vi "DAQ_System.vi"() -> ()   [LabVIEW 2023]
uses:
  Controls/Control 5.ctl
  Controls/Control 4.ctl
  Controls/Queue_Operation_Select.ctl
  Controls/Acquired_Data.ctl
  Controls/State_and_Data.ctl
panel:
  out "Error_Out":errorcluster
  in  "Error_In":errorcluster
  in  "Stop":bool
  out "DAQ_Output":T1
  in  "DAQ_Inputs":T2 caption="DAQ Inputs" {"Analog_In"."Battery_Power" scale=0.0..10.0; "Analog_In"."Power_Consumption" scale=0.0..10.0}
  # "DAQ Simulator"
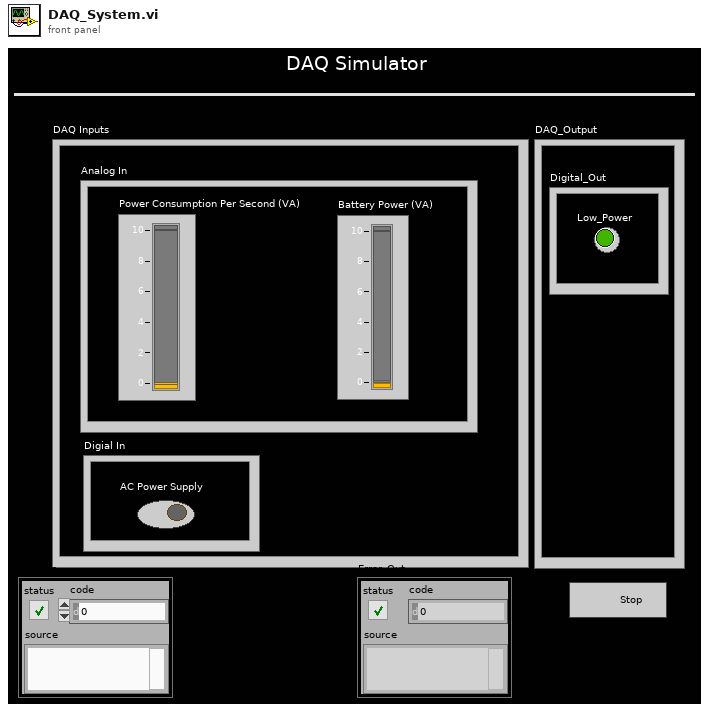
[diagram p1: front panel]
types:
  T1 = typedef "Control 4.ctl" = cluster{"Digital_Out":cluster{"Low_Power":bool}}
  T2 = typedef "Control 5.ctl" = cluster{"Digial_In":cluster{"AC_Power_Supply":bool}, "Analog_In":cluster{"Power_Consumption":dbl, "Battery_Power":dbl}}
  T3 = typedef "Acquired_Data.ctl" = cluster{"Battery_Power":dbl, "Power_Consumption":dbl, "Inverter_Mode":bool}
  T4 = typedef "State_and_Data.ctl" = cluster{"State":string, "Data":variant}
  T5 = cluster{"Low_Power?":bool, "Acquired_Data":T3, "DAQ_Output":T1, "DAQ_Inputs":T2, "Data_In":T4, "Start":bool}
  T6 = enum32{"Invalid", "Standard", "Closed", "Hidden", "Minimized", "Maximized"}
  T7 = typedef "Queue_Operation_Select.ctl" = enum16{"Obtain_Queue", "Enqueue", "Enqueue_First", "Enqueue_N", "Lossy_Enqueue", "Preview", "Queue_Status", "Dequeue", "Flush", "Release_Queue"}
  T8 = cluster{"Power_Consumption":dbl, "Battery_Power":dbl}
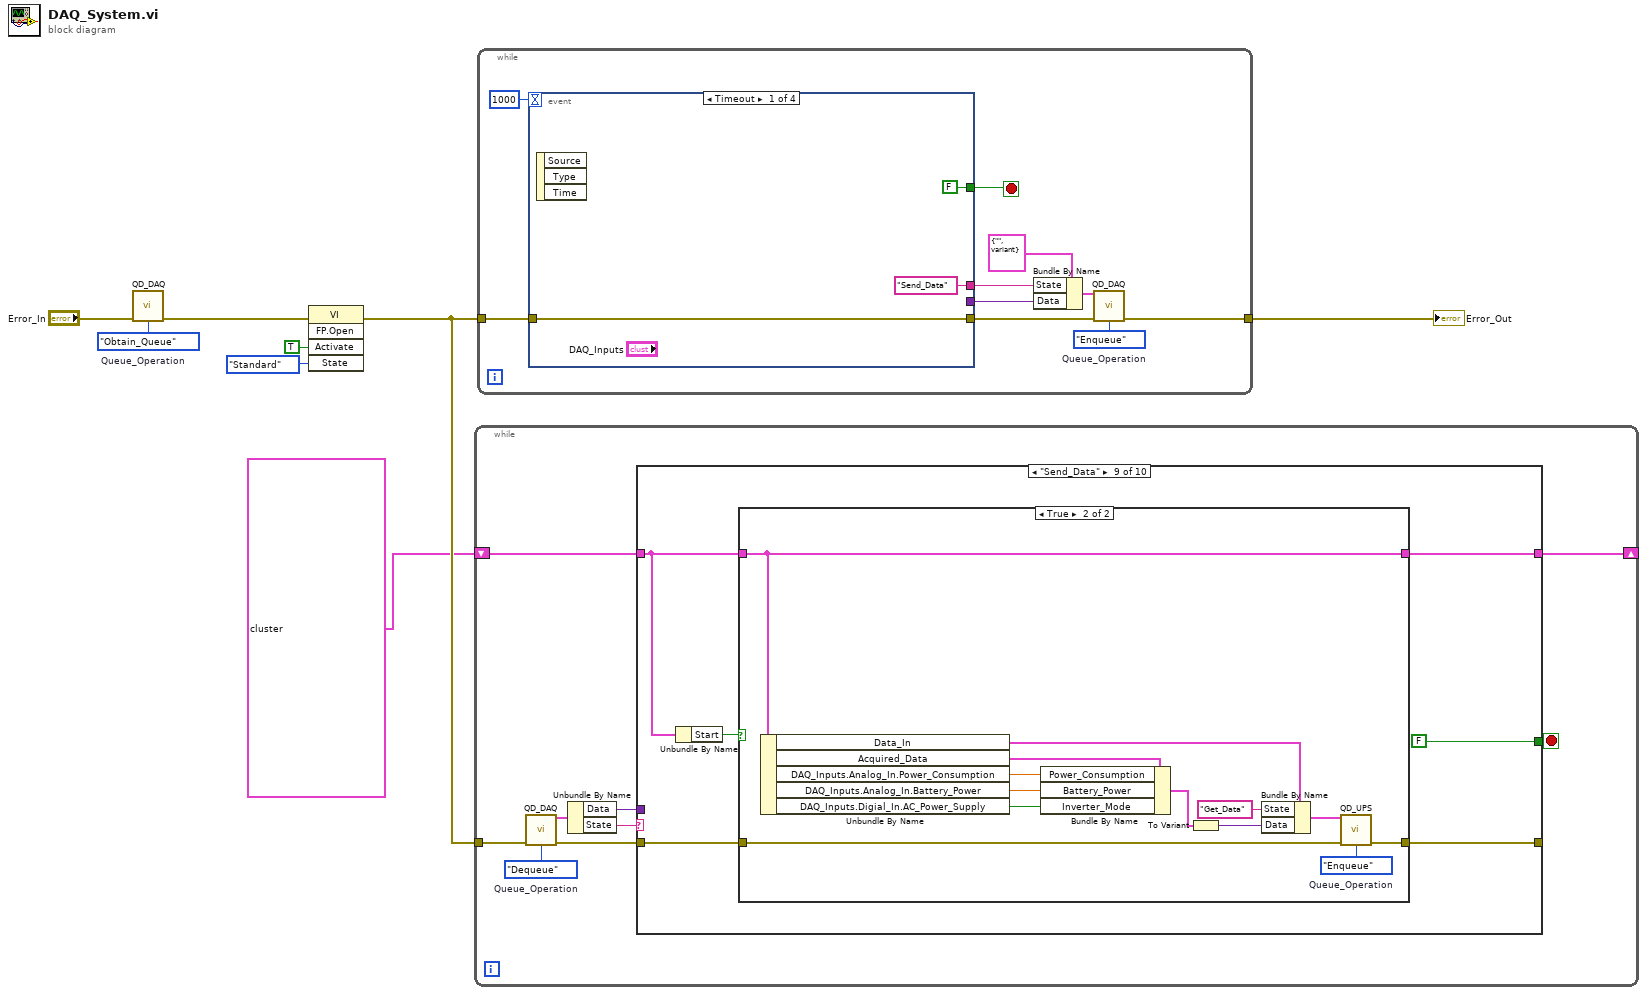
[diagram p0: block diagram]
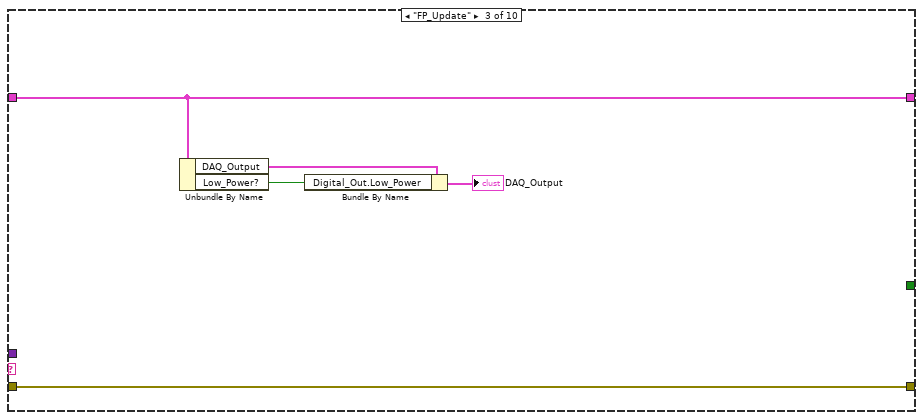
[diagram p4: hidden frame]
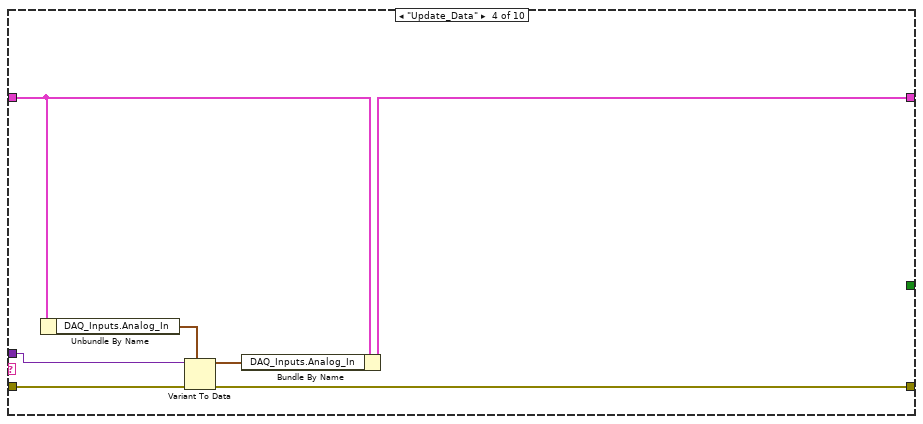
[diagram p5: hidden frame]
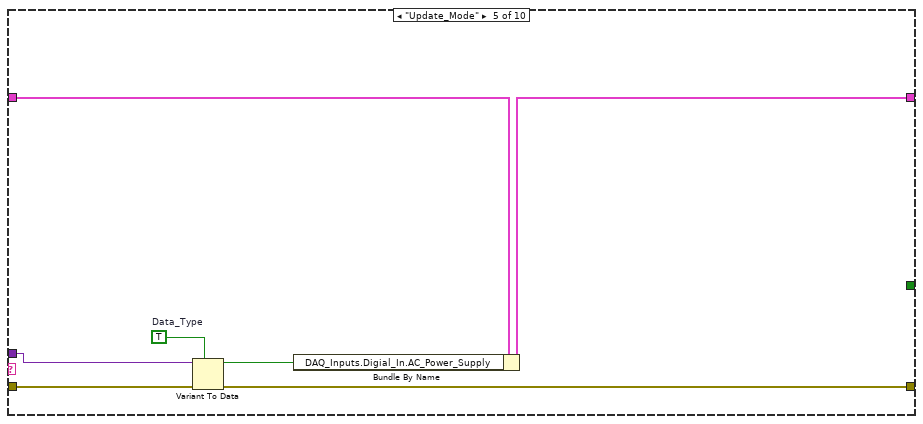
[diagram p6: hidden frame]
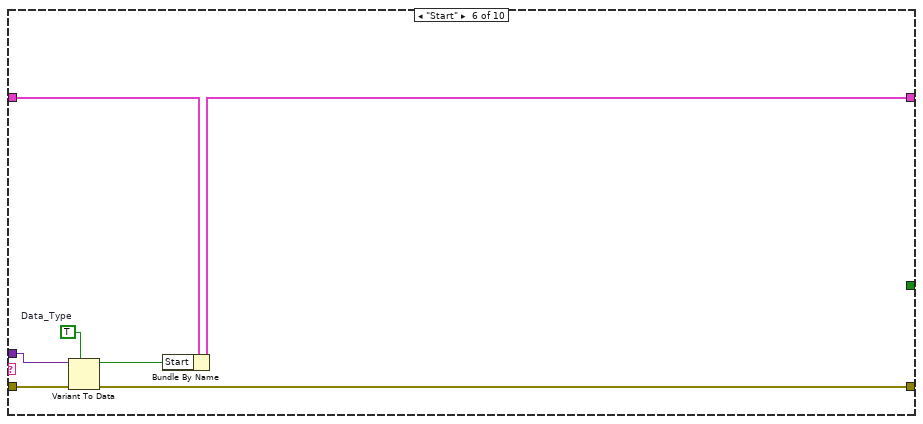
[diagram p7: hidden frame]
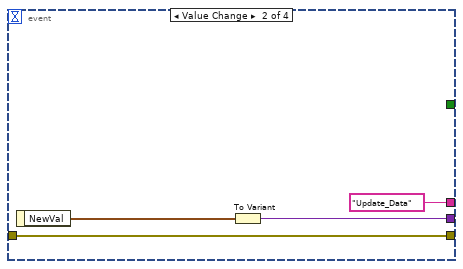
[diagram p12: hidden frame]
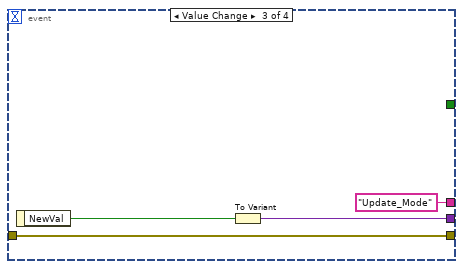
[diagram p13: hidden frame]
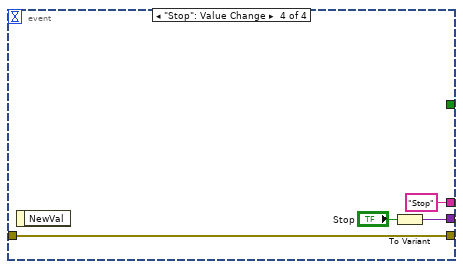
[diagram p14: hidden frame]
diagram:
  w5 = Queue_Operation_Select."Obtain_Queue"  # Queue_Operation
  n1 = call "QD_DAQ.vi"("Error_In"="Error_In", "Queue_Operation"=w5) -> ("Error_Out"=w6:errorcluster)  [unwired: 11 in, 2 out]
  n2 = invoke class="VI" method="FP.Open"(error in=w6, "Activate"=TRUE ("Activate?"), "State"=T6."Standard") -> (error out=w2:errorcluster)  [unwired: 2 in, 4 out]
  n3 = while {
    tunnel: w2 -> [w17]
    shift-right: [w11] -> _
    shift-left: T5 {"Low_Power?"=FALSE, "Acquired_Data"={"Battery_Power"=0.0, "Power_Consumption"=0.0, "Inverter_Mode"=FALSE}, "DAQ_Output"={"Digital_Out"={"Low_Power"=FALSE}}, "DAQ_Inputs"={"Digial_In"={"AC_Power_Supply"=FALSE}, "Analog_In"={"Power_Consumption"=0.0, "Battery_Power"=0.0}}, "Data_In"={"State"="", "Data"=variant}, "Start"=FALSE} -> [w10]
    stop <- w9 stop-if-true
    w15 = Queue_Operation_Select."Dequeue"  # Queue_Operation
    n4 = call "QD_DAQ.vi"("Error_In"=w17, "Queue_Operation"=w15) -> ("Data_Out"=w14:T4, "Error_Out"=w16:errorcluster)  [unwired: 11 in, 1 out]
    n5 = Unbundle By Name(w14) -> ("Data"=w12:variant, "State"=w13:string)
    n6 = case shown="\"Send_Data\"" w13 {
      tunnel: w16 -> [w19 w21 w26 w33 w40 w47 w49 w51 w57 w74]
      tunnel: [w19 w21 w26 w32 w39 w45 w49 w51 w56 w74] -> _
      tunnel: w12 -> [_ _ _ w31 w38 w44 _ _ _ _]
      tunnel: [w18 w20 w25 w28 w35 w42 w48 w50 w55 w73] -> w11
      tunnel: w10 -> [w18 w20 w25 w29 w37 w46 w48 w50 w54 w73]
      tunnel: [_ _ _ _ _ _ _ _ FALSE _] -> w9
      frame Default {
      }
      frame "Initialize" {
      }
      frame "FP_Update" {
        n7 = Unbundle By Name(w25) -> ("DAQ_Output"=w23:T1, "Low_Power?"=w22:bool)
        n8 = Bundle By Name(cluster=w23, "Digital_Out.Low_Power"=w22) -> (→"DAQ_Output":T1)
      }
      frame "Update_Data" {
        n9 = Unbundle By Name(w29) -> ("DAQ_Inputs.Analog_In"=w30:T8)
        n10 = Variant To Data(error in=w33, type=w30, Variant=w31) -> (data=w27:T8, error out=w32:errorcluster)
        n11 = Bundle By Name(cluster=w29, "DAQ_Inputs.Analog_In"=w27) -> (w28:T5)
      }
      frame "Update_Mode" {
        w36 = TRUE  # Data_Type
        n12 = Variant To Data(error in=w40, type=w36, Variant=w38) -> (data=w34:bool, error out=w39:errorcluster)
        n13 = Bundle By Name(cluster=w37, "DAQ_Inputs.Digial_In.AC_Power_Supply"=w34) -> (w35:T5)
      }
      frame "Start" {
        w43 = TRUE  # Data_Type
        n14 = Variant To Data(error in=w47, type=w43, Variant=w44) -> (data=w41:bool, error out=w45:errorcluster)
        n15 = Bundle By Name(cluster=w46, "Start"=w41) -> (w42:T5)
      }
      frame "Stop" {
      }
      frame "Charge_Discharge" {
      }
      frame "Send_Data" {
        n16 = Unbundle By Name(w54) -> ("Start"=w53:bool)
        n17 = case shown="True" w53 {
          tunnel: w57 -> [w58 w72]
          tunnel: [w58 w71] -> w56
          tunnel: [w59 w66] -> w55
          tunnel: w54 -> [w59 w66]
          frame False {
          }
          frame True {
            w70 = Queue_Operation_Select."Enqueue"  # Queue_Operation
            n18 = Unbundle By Name(w66) -> ("Data_In"=w65:T4, "Acquired_Data"=w64:T3, "DAQ_Inputs.Analog_In.Power_Consumption"=w63:dbl, "DAQ_Inputs.Analog_In.Battery_Power"=w62:dbl, "DAQ_Inputs.Digial_In.AC_Power_Supply"=w61:bool)
            n19 = Bundle By Name(cluster=w64, "Power_Consumption"=w63, "Battery_Power"=w62, "Inverter_Mode"=w61) -> (w60:T3)
            n20 = To Variant(anything=w60) -> (Variant=w68:variant)
            n21 = Bundle By Name(cluster=w65, "State"="Get_Data", "Data"=w68) -> (w69:T4)
            n22 = call "QD_UPS.vi"("State_and_Data_In"=w69, "Error_In"=w72, "Queue_Operation"=w70) -> ("Error_Out"=w71:errorcluster)  [unwired: 11 in, 1 out]
          }
        }
      }
      frame "Error" {
      }
    }
  }
  n23 = while {
    tunnel: w2 -> [w84]
    tunnel: [w82] -> w8
    stop <- w76 stop-if-true
    w81 = Queue_Operation_Select."Enqueue"  # Queue_Operation
    n24 = event shown="[0] Timeout" {
      selector: _ -> [_ _ _ _]
      dyn-events: _ -> [_ _ _ _]
      timeout: 1000 -> [_ _ _ _]
      tunnel: w84 -> [w87 w91 w95 w99]
      tunnel: [w87 w91 w95 w99] -> w83
      tunnel: ["Send_Data" ("State") "Update_Data" ("State") "Update_Mode" ("State") "Stop" ("State")] -> w78
      tunnel: [_ w88 w93 w97] -> w77
      tunnel: [FALSE _ _ _] -> w76
      event Timeout {
        n25 = event-data() -> ()  [unwired: 1 in, 3 out]
      }
      event Value Change {
        n26 = event-data() -> ("NewVal"=w89:T8)  [unwired: 1 in]
        n27 = To Variant(anything=w89) -> (Variant=w88:variant)
      }
      event Value Change {
        n28 = event-data() -> ("NewVal"=w94:bool)  [unwired: 1 in]
        n29 = To Variant(anything=w94) -> (Variant=w93:variant)
      }
      event "Stop": Value Change {
        n30 = event-data() -> ()  [unwired: 1 in, 1 out]
        n31 = To Variant(anything="Stop") -> (Variant=w97:variant)
      }
    }
    n32 = Bundle By Name(cluster=T4 {"State"="", "Data"=variant} ("Data_In"), "State"=w78, "Data"=w77) -> (w80:T4)
    n33 = call "QD_DAQ.vi"("Data_In"=w80, "Error_In"=w83, "Queue_Operation"=w81) -> ("Error_Out"=w82:errorcluster)  [unwired: 10 in, 2 out]
  }
  "Error_Out" <- w8
